vi "BASE-Julian Code.vi"() -> (0 "Long Date":string, 1 "Short Date":string, 2 "Shift":string, 3 "Julian Code":string, 4 "Long time with :":string, 5 "Long date with /":string)   [LabVIEW 2017]
panel:
  out "Shift 2":string
  out "date/time string":string
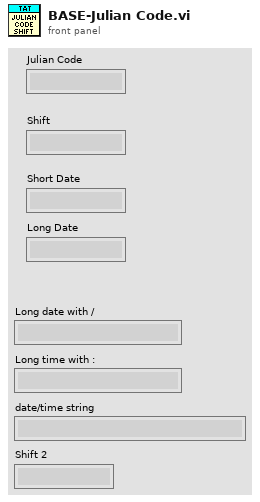
[diagram p1: front panel]
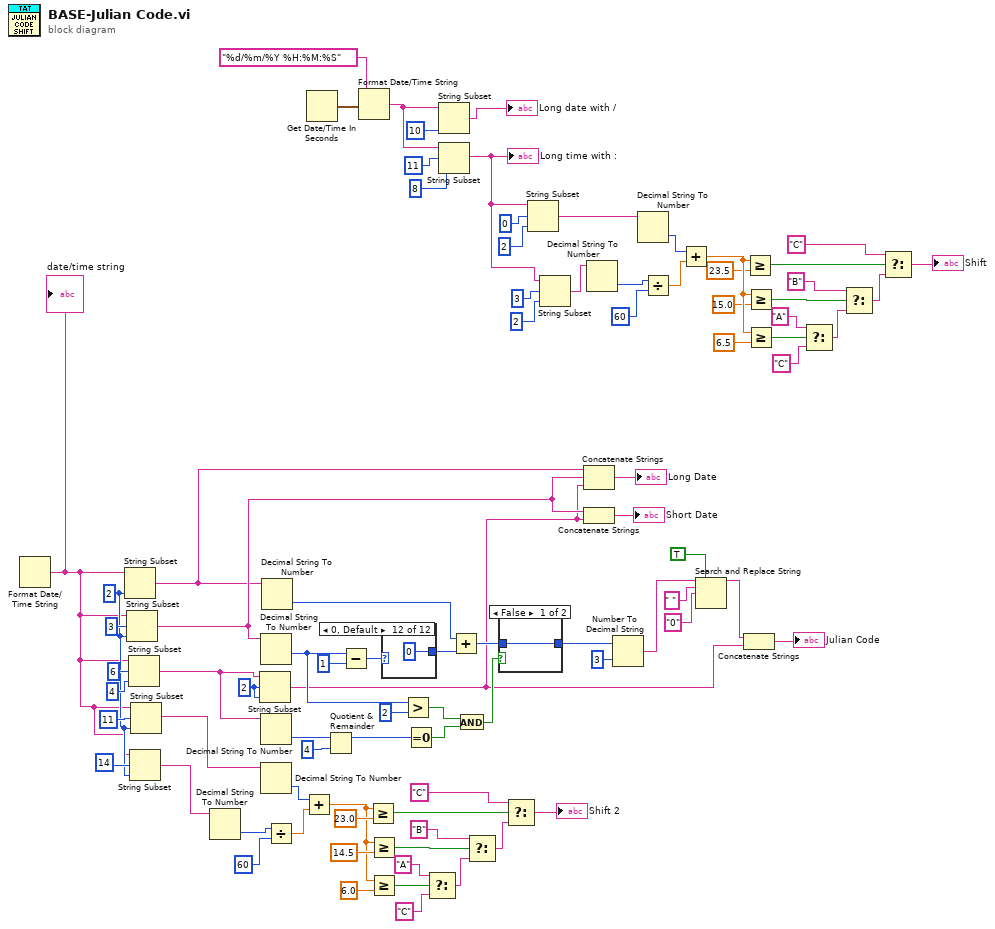
[diagram p0: block diagram]
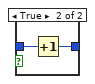
[diagram p2: hidden frame]
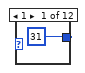
[diagram p3: hidden frame]
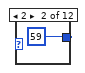
[diagram p4: hidden frame]
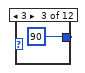
[diagram p5: hidden frame]
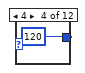
[diagram p6: hidden frame]
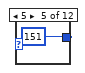
[diagram p7: hidden frame]
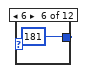
[diagram p8: hidden frame]
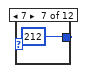
[diagram p9: hidden frame]
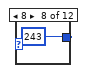
[diagram p10: hidden frame]
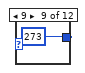
[diagram p11: hidden frame]
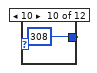
[diagram p12: hidden frame]
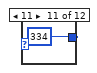
[diagram p13: hidden frame]
diagram:
  w60 = 2 ("length (rest)")
  w87 = 2 ("offset (0)")
  n1 = Format Date/Time String() -> (date/time string=w31:string)  [unwired: 3 in]
  "date/time string" <- w31
  n2 = String Subset(string=w31, length (rest)=w60) -> (substring=w35:string)  [unwired: 1 in]
  n3 = String Subset(string=w31, offset (0)=3, length (rest)=w60) -> (substring=w37:string)
  n4 = String Subset(string=w31, offset (0)=6, length (rest)=4 ("length (rest)")) -> (substring=w74:string)
  n5 = String Subset(string=w31, offset (0)=14, length (rest)=w60) -> (substring=w59:string)
  n6 = String Subset(string=w31, offset (0)=11, length (rest)=w60) -> (substring=w53:string)
  n7 = Decimal String To Number(string=w59) -> (number=w58:i32)  [unwired: 2 in, 1 out]
  n8 = String Subset(string=w74, offset (0)=w87, length (rest)=w87) -> (substring=w36:string)
  n9 = Decimal String To Number(string=w37) -> (number=w46:i32)  [unwired: 2 in, 1 out]
  n10 = Decimal String To Number(string=w74) -> (number=w86:i32)  [unwired: 2 in, 1 out]
  n11 = Decimal String To Number(string=w53) -> (number=w56:i32)  [unwired: 2 in, 1 out]
  n12 = Decimal String To Number(string=w35) -> (number=w81:i32)  [unwired: 2 in, 1 out]
  n13 = Divide(x=w58, y=60) -> (x/y=w55:dbl)
  n14 = Add(x=w56, y=w55) -> (x+y=w54:dbl)
  n15 = Get Date/Time In Seconds() -> (seconds since 1Jan1904=w3:timestamp)
  n16 = Quotient & Remainder(x=w86, y=4) -> (x-y*floor(x/y)=w84:i32)  [unwired: 1 out]
  n17 = Subtract(x=w46, y=1) -> (x-y=w82:i32)
  n18 = Format Date/Time String(time format string (%c)="%d/%m/%Y %H:%M:%S", seconds (now)=w3) -> (date/time string=w6:string)  [unwired: 1 in]
  n19 = Greater Or Equal?(x=w54, y=23.0) -> (x >= y?=w70:bool)
  n20 = Greater Or Equal?(x=w54, y=14.5) -> (x >= y?=w63:bool)
  n21 = Greater Or Equal?(x=w54, y=6.0) -> (x >= y?=w65:bool)
  n22 = case shown="0, Default" w82 {
    tunnel: [31 ("y") 59 ("y") 90 ("y") 120 ("y") 151 ("y") 181 ("y") 212 ("y") 243 ("y") 273 ("y") 308 ("y") 334 ("y") 0 ("y")] -> w80
    frame 1 {
    }
    frame 2 {
    }
    frame 3 {
    }
    frame 4 {
    }
    frame 5 {
    }
    frame 6 {
    }
    frame 7 {
    }
    frame 8 {
    }
    frame 9 {
    }
    frame 10 {
    }
    frame 11 {
    }
    frame 0, Default {
    }
  }
  n23 = Greater?(x=w46, y=2) -> (0:w44:bool)
  n24 = Equal To 0?(x=w84) -> (x = 0?=w43:bool)
  n25 = Select(t="A", s=w65, f="C") -> (s? t:f=w67:string)
  n26 = String Subset(string=w6, length (rest)=10 ("length (rest)")) -> (substring=→"Long date with /":string)  [unwired: 1 in]
  n27 = String Subset(string=w6, offset (0)=11 ("length (rest)"), length (rest)=8 ("length (rest)")) -> (substring=w4:string)
  "Long time with :" <- w4
  n28 = Add(x=w81, y=w80) -> (x+y=w48:i32)
  n29 = And(x=w44, y=w43) -> (x .and. y?=w42:bool)
  n30 = Select(t="B", s=w63, f=w67) -> (s? t:f=w68:string)
  n31 = case shown="False" w42 {
    tunnel: w48 -> [w100 w102]
    tunnel: [w100 w101] -> w47
    frame False {
    }
    frame True {
      n32 = Increment(x=w102) -> (x+1=w101:i32)
    }
  }
  n33 = Select(t="C", s=w70, f=w68) -> (s? t:f=→"Shift 2":string)
  n34 = String Subset(string=w4, offset (0)=0 ("length (rest)"), length (rest)=2 ("length (rest)")) -> (substring=w9:string)
  n35 = String Subset(string=w4, offset (0)=3 ("length (rest)"), length (rest)=2 ("length (rest)")) -> (substring=w5:string)
  n36 = Concatenate Strings(w35, w37, w36) -> (→"Long Date":string)
  n37 = Concatenate Strings(w37, w36) -> (→"Short Date":string)
  n38 = Decimal String To Number(string=w5) -> (number=w24:i32)  [unwired: 2 in, 1 out]
  n39 = Number To Decimal String(number=w47, width (-)=i16 3) -> (decimal integer string=w51:string)
  n40 = Decimal String To Number(string=w9) -> (number=w26:i32)  [unwired: 2 in, 1 out]
  n41 = Divide(x=w24, y=60) -> (x/y=w27:dbl)
  n42 = Add(x=w26, y=w27) -> (x+y=w28:dbl)
  n43 = Search and Replace String(replace all?=TRUE ("replace all? (F)"), input string=w51, search string=" ", replace string="0" ("replace string (\"\")")) -> (result string=w41:string)  [unwired: 4 in, 3 out]
  n44 = Concatenate Strings(w41, w36) -> (→"Julian Code":string)
  n45 = Greater Or Equal?(x=w28, y=23.5) -> (x >= y?=w15:bool)
  n46 = Greater Or Equal?(x=w28, y=15.0) -> (x >= y?=w22:bool)
  n47 = Greater Or Equal?(x=w28, y=6.5) -> (x >= y?=w20:bool)
  n48 = Select(t="A", s=w20, f="C") -> (s? t:f=w18:string)
  n49 = Select(t="B", s=w22, f=w18) -> (s? t:f=w17:string)
  n50 = Select(t="C", s=w15, f=w17) -> (s? t:f=→"Shift":string)
